vi "Get Source.vi"(8 "Error In":errorcluster) -> (0 "Error Out":errorcluster, 3 "Source":string)   [LabVIEW 2014, in "LV-Logger.lvlib"]
uses:
  LV-Logger.lvlib
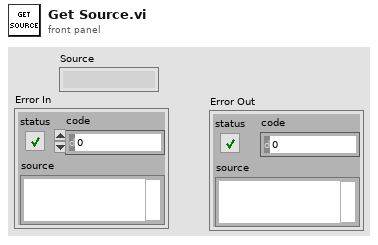
[diagram p1: front panel]
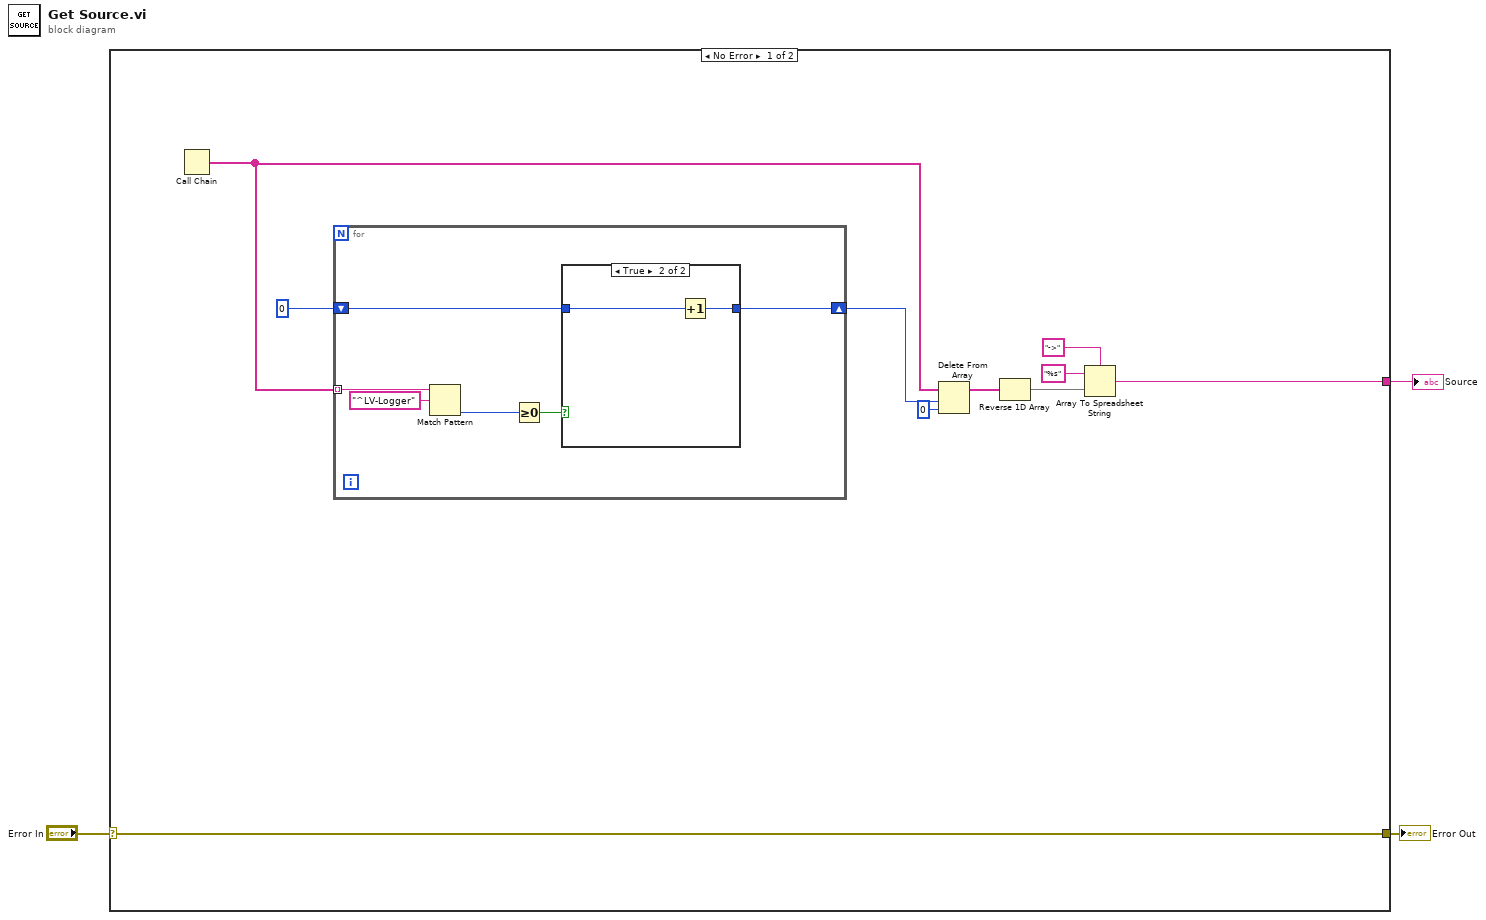
[diagram p0: block diagram]
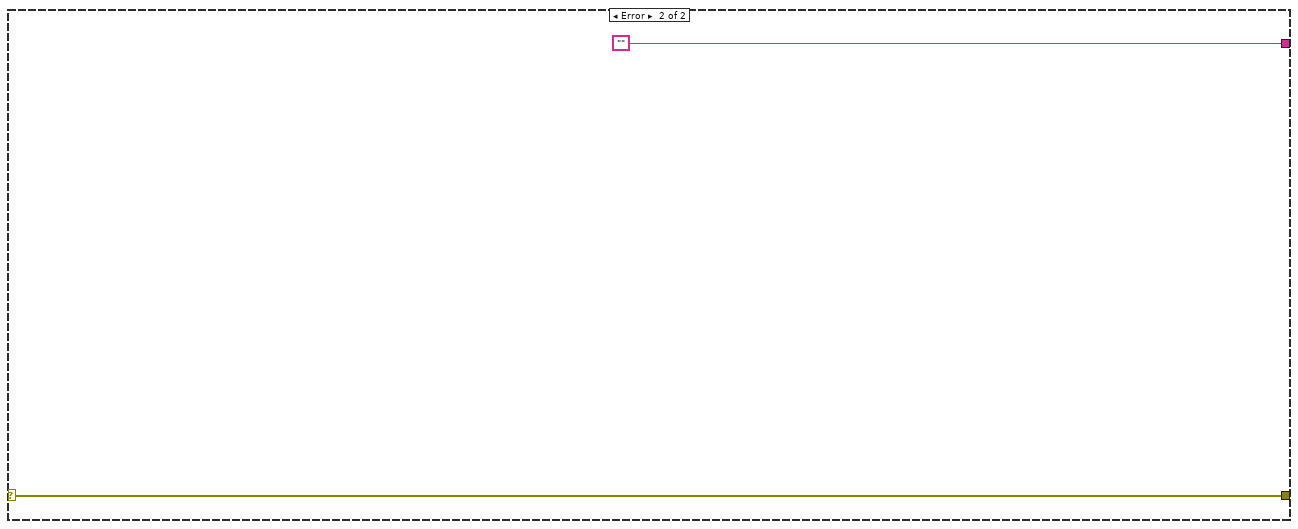
[diagram p3: hidden frame]
diagram:
  n1 = case shown="No Error" "Error In" {
    selector: "Error In" -> [w9 w23]
    tunnel: [w10 ""] -> w3
    tunnel: [w9 w23] -> w1
    frame No Error {
      n2 = Call Chain() -> (call chain=w7:string[])
      n3 = for {
        tunnel: w7 -> [w19] mode=indexing
        shift-right: [w14] -> w6
        shift-left: 0 -> [w15]
        n4 = Match Pattern(string=w19, regular expression="^LV-Logger") -> (offset past match=w17:i32)  [unwired: 1 in, 3 out]
        n5 = Greater Or Equal To 0?(x=w17) -> (x >= 0?=w16:bool)
        n6 = case shown="True" w16 {
          tunnel: w15 -> [w20 w22]
          tunnel: [w20 w21] -> w14
          frame False {
          }
          frame True {
            n7 = Increment(x=w22) -> (x+1=w21:i32)
          }
        }
      }
      n8 = Delete From Array(array=w7, length=w6, index=0) -> (array with subset deleted=w4:string[])  [unwired: 1 out]
      n9 = Reverse 1D Array(array=w4) -> (reversed array=w13:string[])
      n10 = Array To Spreadsheet String(delimiter (Tab)="->", array=w13, 3:"%s" ("format string")) -> (spreadsheet string=w10:string)
    }
    frame Error {
    }
  }
  "Source" <- w3
  "Error Out" <- w1
